vi "Ping Actor.vi"(8 "error in (no error)":errorcluster, 10 "Actor":refnum<class "Message Enqueuer.lvclass">, 11 "Actor Monitor New in":refnum<class "Actor Monitor.lvclass">) -> (0 "error out":errorcluster, 3 "Actor Monitor New out":refnum<class "Actor Monitor.lvclass">)   [LabVIEW 2017, in "MGI-Monitored Actor Core.lvlib" / "Actor Monitor.lvclass"]
doc: "Sends a ping message to the actor\n\nCopyright: MGI 2016\nAuthor: Derek Trepanier"
uses:
  Actor Monitor.lvclass
  <vilib>/ActorFramework/Message Enqueuer/Message Enqueuer.lvclass
  Actor Monitor.lvclass/Actor Monitor.ctl
  Monitored Actor/Monitored Actor Messages/Ping Msg/Ping Msg.lvclass
  Monitor Data/Monitor Data.lvclass
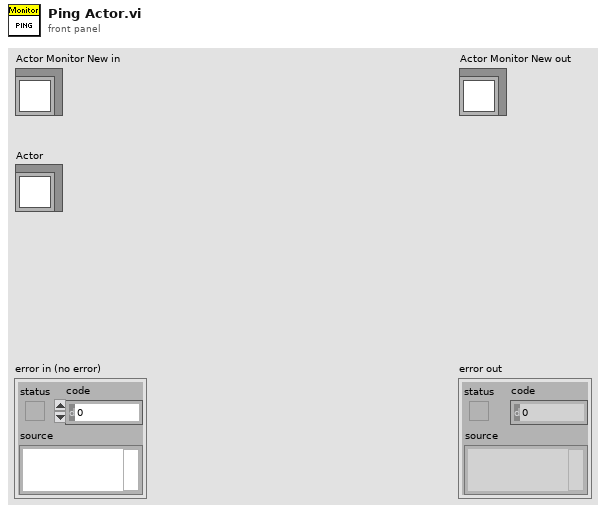
[diagram p1: front panel]
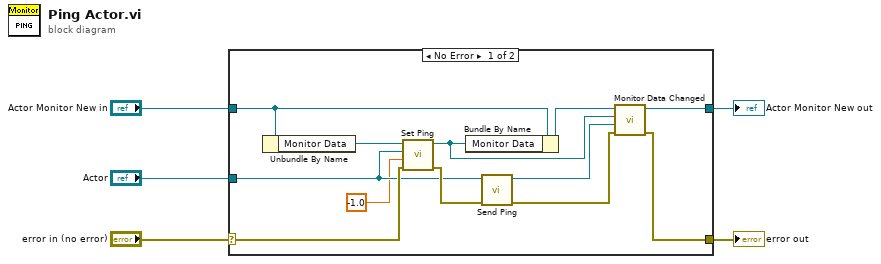
[diagram p0: block diagram]
diagram:
  n1 = case shown="No Error" "error in (no error)" {
    selector: "error in (no error)" -> [w13 w19]
    tunnel: [w7 w19] -> w4
    tunnel: [w10 w18] -> w2
    tunnel: "Actor Monitor New in" -> [w17 w18]
    tunnel: "Actor" -> [w12 _]
    frame No Error {
      n2 = Unbundle By Name(w17) -> ("Monitor Data"=w16:refnum<class "Monitor Data.lvclass">)
      n3 = call "Set Ping.vi"("error in (no error)"=w13, "Ping Duration"=-1.0, "Actor's Self Q"=w12, "Monitor Data in"=w16) -> ("error out"=w14:errorcluster, "Monitor Data out"=w9:refnum<class "Monitor Data.lvclass">)  [unwired: 6 in]
      n4 = Bundle By Name(cluster=w17, "Monitor Data"=w9) -> (w15:refnum<class "Actor Monitor.lvclass">)
      n5 = call "Send Ping.vi"("error in (no error)"=w14, "Message Enqueuer in"=w12) -> ("error out"=w8:errorcluster, "Message Enqueuer out"=w6:refnum<class "Message Enqueuer.lvclass">)  [unwired: 8 in]
      n6 = call-dynamic "Monitor Data Changed.vi"("error in (no error)"=w8, "Changed Actor's Q"=w6, "Monitor Data"=w9, "Actor Monitor New in"=w15) -> ("error out"=w7:errorcluster, "Actor Monitor New out"=w10:refnum<class "Actor Monitor.lvclass">)  [unwired: 6 in]
    }
    frame Error {
    }
  }
  "error out" <- w4
  "Actor Monitor New out" <- w2
